vi "dfd_DFXP Mul (ss).vi"(7 "op params":T5={"source"=0, "is floating?"=FALSE, "o-mode"=enum."Wrap", "q-mode"=enum."Truncation", "wl"=1, "high limit"=0, "low limit"=0, "iwl"=0, "sign?"=TRUE} {"source" items=["Coef a/k"=0, "Coef b/v"=7, "Input"=1, "Output"=2, "Multiplicand"=3, "Product"=4, "Sum"=5, "Delay"=6, "Gain"=8]}, 8 "filtering statistics in":T4(array[cluster]) {"statistics information"."min value" format="%.2f"; "statistics information"."max value" format="%.2f"; "Quantizer Source" items=["Coefficients a/k"=0, "Coefficients b/v"=7, "Input"=1, "Output"=2, "Multiplicand"=3, "Product"=4, "Sum"=5, "Delay"=6]}, 9 "Value in 2":T1={"value"=0, "wl"=0, "iwl"=0, "Signed"=TRUE} {"value" format="%.0x"}, 10 "Value in":T1={"value"=0, "wl"=0, "iwl"=0, "Signed"=TRUE} {"value" format="%.0x"}) -> (0 "filtering statistics out":T4(array[cluster]) {"statistics information"."min value" format="%.2f"; "statistics information"."max value" format="%.2f"; "Quantizer Source" items=["Coefficients a/k"=0, "Coefficients b/v"=7, "Input"=1, "Output"=2, "Multiplicand"=3, "Product"=4, "Sum"=5, "Delay"=6]}, 2 "Value out":T1={"value"=0, "wl"=0, "iwl"=0, "Signed"=TRUE} {"value" format="%.0x"})   [LabVIEW 2017, in "NI_DigFilter_FXP.lvlib"]
uses:
  <vilib>/addons/Digital Filter Design/NI_DigFilter_FXP.lvlib
  <vilib>/addons/Digital Filter Design/_Objects.llb/dfd_DFXP Data Type (scaler).ctl
  <vilib>/addons/Digital Filter Design/_Objects.llb/dfd_DFXP Data Type 128bits (scaler).ctl
  <vilib>/addons/Digital Filter Design/_Objects.llb/DFD Quantization Sources.ctl
  <vilib>/addons/Digital Filter Design/_Objects.llb/DFD FXP Statistics Data.ctl
  <vilib>/addons/Digital Filter Design/_Objects.llb/dfd_DFXP Operation Parameter.ctl
  <vilib>/addons/Digital Filter Design/_Objects.llb/dfd_Internal Quantization Srcs.ctl
  <vilib>/addons/Digital Filter Design/NI_DigFilterLicensed.lvlib
panel:
  in  "Value out type":T1={"value"=0, "wl"=0, "iwl"=0, "Signed"=TRUE} {"value" format="%.0x"}
  in  "Value out type":T7 {"Low 64" format="%.0x"; "High 64" format="%.0x"}
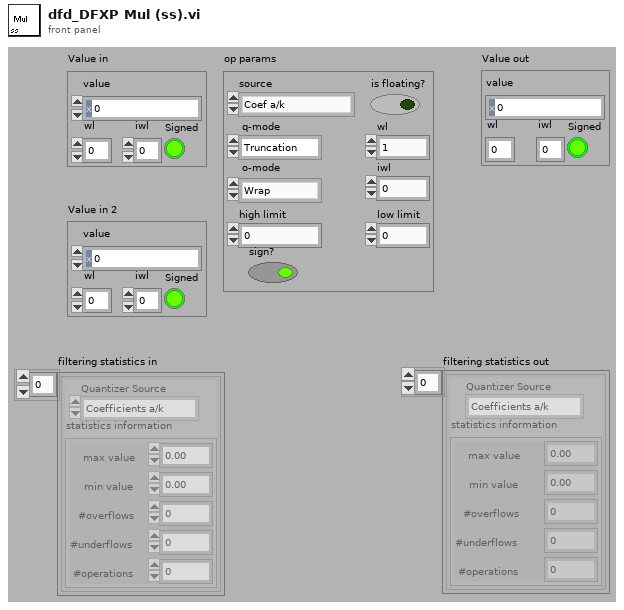
[diagram p1: front panel]
types:
  T1 = typedef "dfd_DFXP Data Type (scaler).ctl" = cluster{"value":i64, "wl":i16, "iwl":i16, "Signed":bool}
  T2 = typedef "NI_DigFilterLicensed.lvlib/DFD Quantization Sources.ctl" = u16
  T3 = typedef "NI_DigFilterLicensed.lvlib/DFD FXP Statistics Data.ctl" = cluster{"max value":ext, "min value":ext, "#overflows":i32, "#underflows":i32, "#operations":i32}
  T4 = cluster{"Quantizer Source":T2, "statistics information":T3}[]
  T5 = typedef "dfd_DFXP Operation Parameter.ctl" = cluster{"source":T6, "is floating?":bool, "o-mode":enum16{"Saturation", "Wrap"}, "q-mode":enum16{"Nearest", "Truncation"}, "wl":i16, "high limit":i64, "low limit":i64, "iwl":i16, "sign?":bool}
  T6 = typedef "NI_DigFilterLicensed.lvlib/dfd_Internal Quantization Srcs.ctl" = u16
  T7 = typedef "dfd_DFXP Data Type 128bits (scaler).ctl" = cluster{"Low 64":u64, "High 64":i64, "wl":i16, "iwl":i16}
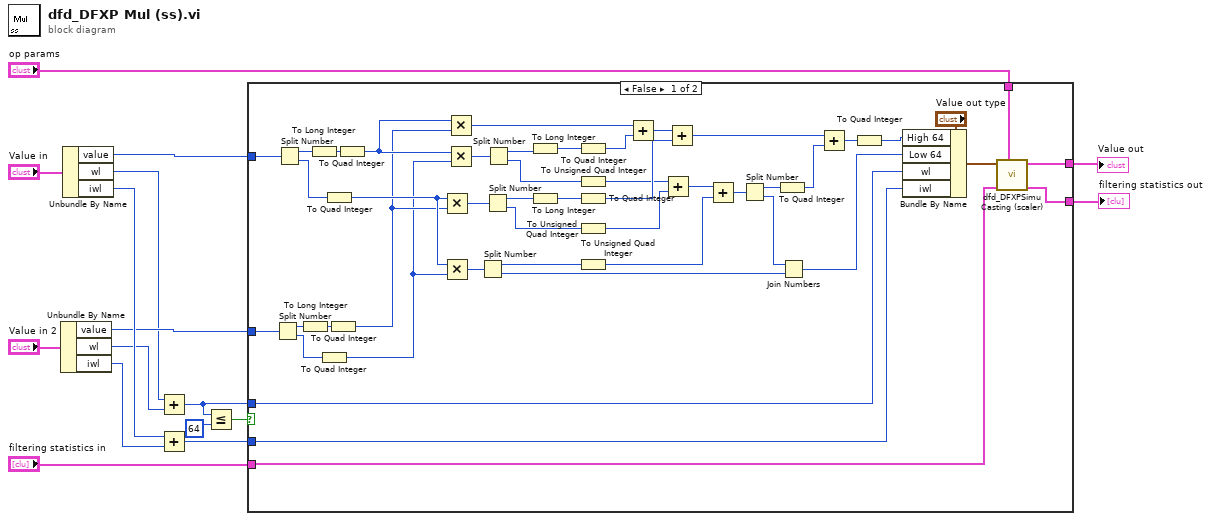
[diagram p0: block diagram]
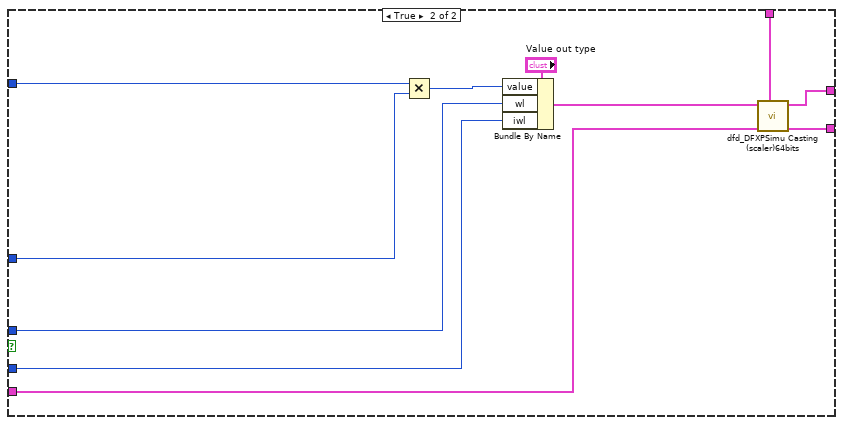
[diagram p2: hidden frame]
diagram:
  n1 = Unbundle By Name("Value in 2") -> ("value"=w2:i64, "wl"=w9:i16, "iwl"=w10:i16)
  n2 = Unbundle By Name("Value in") -> ("value"=w3:i64, "wl"=w1:i16, "iwl"=w12:i16)
  n3 = Add(x=w1, y=w9) -> (x+y=w11:i16)
  n4 = Add(x=w12, y=w10) -> (x+y=w8:i16)
  n5 = Less Or Equal?(x=w11, y=i16 64) -> (x <= y?=w15:bool)
  n6 = case shown="False" w15 {
    tunnel: w11 -> [w37 w66]
    tunnel: w8 -> [w36 w65]
    tunnel: "filtering statistics in" -> [w34 w72]
    tunnel: "op params" -> [w33 w70]
    tunnel: [w32 w69] -> w5
    tunnel: [w31 w71] -> w4
    tunnel: w3 -> [w25 w67]
    tunnel: w2 -> [w19 w68]
    frame False {
      n7 = Split Number(x=w19) -> (hi(x)=w22:u32, lo(x)=w20:u32)
      n8 = Split Number(x=w25) -> (hi(x)=w28:u32, lo(x)=w26:u32)
      n9 = To Long Integer(number=w22) -> (32bit integer=w21:i32)
      n10 = To Long Integer(number=w28) -> (32bit integer=w27:i32)
      n11 = To Quad Integer(1:w20) -> (0:w17:i64)
      n12 = To Quad Integer(1:w26) -> (0:w23:i64)
      n13 = To Quad Integer(1:w21) -> (0:w18:i64)
      n14 = To Quad Integer(1:w27) -> (0:w24:i64)
      n15 = Multiply(x=w23, y=w18) -> (x*y=w60:i64)
      n16 = Multiply(x=w23, y=w17) -> (x*y=w59:i64)
      n17 = Multiply(x=w24, y=w18) -> (x*y=w44:i64)
      n18 = Multiply(x=w24, y=w17) -> (x*y=w61:i64)
      n19 = Split Number(x=w59) -> (hi(x)=w50:u32, lo(x)=w46:u32)
      n20 = Split Number(x=w60) -> (hi(x)=w42:u32, lo(x)=w55:u32)
      n21 = Split Number(x=w61) -> (hi(x)=w43:u32, lo(x)=w56:u32)
      n22 = To Long Integer(number=w43) -> (32bit integer=w40:i32)
      n23 = To Long Integer(number=w42) -> (32bit integer=w41:i32)
      n24 = To Quad Integer(1:w40) -> (0:w58:i64)
      n25 = To Unsigned Quad Integer(1:w56) -> (0:w54:u64)
      n26 = To Quad Integer(1:w41) -> (0:w57:i64)
      n27 = To Unsigned Quad Integer(1:w55) -> (0:w53:u64)
      n28 = To Unsigned Quad Integer(1:w50) -> (0:w51:u64)
      n29 = Add(x=w44, y=w58) -> (x+y=w63:i64)
      n30 = Add(x=w54, y=w53) -> (x+y=w52:u64)
      n31 = Add(x=w63, y=w57) -> (x+y=w62:i64)
      n32 = Add(x=w52, y=w51) -> (x+y=w48:u64)
      n33 = Split Number(x=w48) -> (hi(x)=w47:u32, lo(x)=w45:u32)
      n34 = To Quad Integer(1:w47) -> (0:w49:i64)
      n35 = Join Numbers(hi=w45, lo=w46) -> ((hi.lo)=w29:u64)
      n36 = Add(x=w62, y=w49) -> (x+y=w30:i64)
      n37 = To Quad Integer(1:w30) -> (0:w38:i64)
      n38 = Bundle By Name(cluster="Value out type", "High 64"=w38, "Low 64"=w29, "wl"=w37, "iwl"=w36) -> (w35:T7)
      n39 = call <vilib>:"dfd_DFXPSimu Casting (scaler).vi"("op params"=w33, "filtering statistics in"=w34, "Value in"=w35) -> ("filtering statistics out"=w31:T4, "Value out"=w32:T1)  [unwired: 1 in, 6 out]
    }
    frame True {
      n40 = Multiply(x=w67, y=w68) -> (x*y=w74:i64)
      n41 = Bundle By Name(cluster="Value out type", "value"=w74, "wl"=w66, "iwl"=w65) -> (w73:T1)
      n42 = call <vilib>:"dfd_DFXPSimu Casting (scaler)64bits.vi"("op params"=w70, "filtering statistics in"=w72, "Value in"=w73) -> ("filtering statistics out"=w71:T4, "Value out"=w69:T1)  [unwired: 1 in, 6 out]
    }
  }
  "Value out" <- w5
  "filtering statistics out" <- w4
